vi "main.vi"(0 "x":dbl, 5 "y":dbl) -> (4 "x+y":dbl)   [LabVIEW 2018]
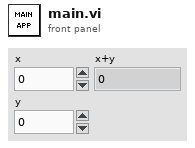
[diagram p1: front panel]
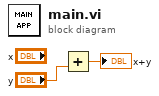
[diagram p0: block diagram]
diagram:
  n1 = Add(y="y") -> (x+y=→"x+y":dbl)  [unwired: 1 in]
